vi "stateAction.vi"(8 "error in (no error)":errorcluster, 11 "Context In":refnum<class "Context.lvclass">) -> (0 "error out":errorcluster, 3 "Context Out":refnum<class "Context.lvclass">)   [LabVIEW 2020, in "Context.lvclass"]
doc: "This method is responsible for calling the State Action and Transition and both of them will dinamy dispatch based on the State subclass contained in Context."
uses:
  Context.lvclass
  Context.lvclass/Context.ctl
  OOP States/State/State.lvclass
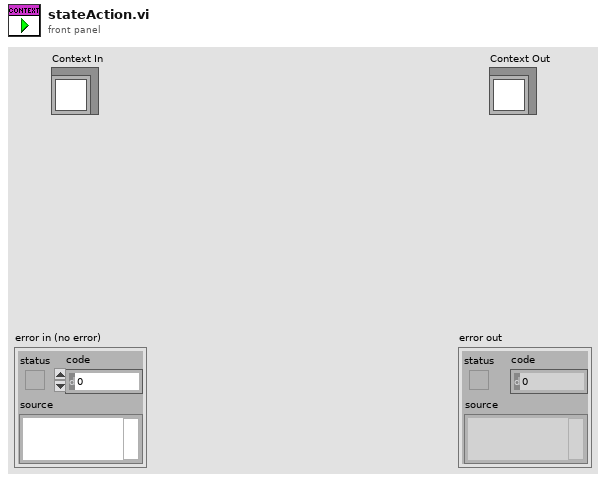
[diagram p1: front panel]
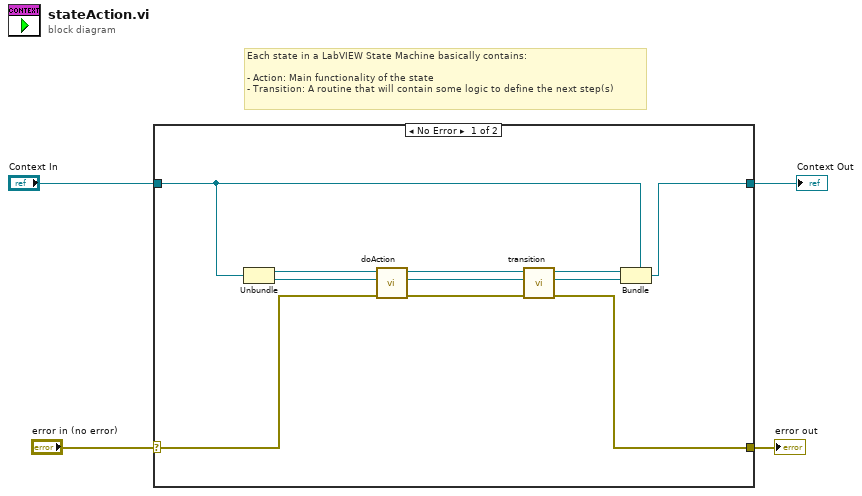
[diagram p0: block diagram]
diagram:
  # "Each state in a LabVIEW State Machine basically contains:\n\n- Action: Main functionality of the state\n- Transition: A routine that will contain some logic to define the next step(s)"
  n1 = case shown="No Error" "error in (no error)" {
    selector: "error in (no error)" -> [w15 w17]
    tunnel: [w14 w17] -> w3
    tunnel: [w5 w16] -> w1
    tunnel: "Context In" -> [w6 w16]
    frame No Error {
      n2 = Unbundle(w6) -> (w12:refnum<class "State.lvclass">, w10:refnum<class "ContextData.lvclass">)
      n3 = call-dynamic "doAction.vi"("error in (no error)"=w15, "ContextData"=w10, "State in"=w12) -> ("error out"=w13:errorcluster, "ContextData Out"=w8:refnum<class "ContextData.lvclass">, "State out"=w11:refnum<class "State.lvclass">)  [unwired: 6 in]
      n4 = call-dynamic "transition.vi"("error in (no error)"=w13, "ContextData In"=w8, "Current State"=w11) -> ("error out"=w14:errorcluster, "ContextData Out"=w7:refnum<class "ContextData.lvclass">, "Next State"=w9:refnum<class "State.lvclass">)  [unwired: 6 in]
      n5 = Bundle(cluster=w6, w9, w7) -> (w5:refnum<class "Context.lvclass">)
    }
    frame Error {
    }
  }
  "error out" <- w3
  "Context Out" <- w1
